vi "Create Template Copy.vi"(8 "error in":errorcluster) -> (0 "error out":errorcluster, 3 "vi refnum":refnum<vi>)   [LabVIEW 2021, in "MeasurementClient Editor.lvlib"]
uses:
  MeasurementClient Editor.lvlib
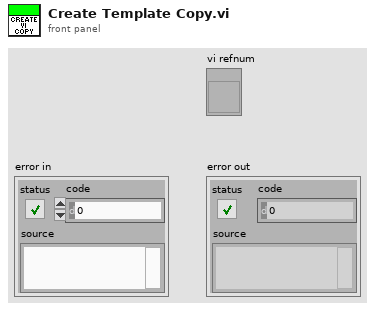
[diagram p1: front panel]
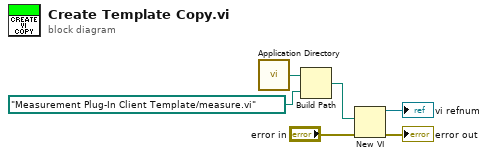
[diagram p0: block diagram]
diagram:
  n1 = call <vilib>:"Application Directory.vi"() -> ("Application Directory"=w3:path)
  n2 = Build Path(base path=w3, name or relative path=path "Measurement Plug-In Client Template/measure.vi") -> (appended path=w1:path)
  n3 = New VI(8:"error in", 10:w1) -> (0:→"error out":errorcluster, 3:→"vi refnum":refnum<vi>)  [unwired: 5 in]
